vi "沿线段检测边沿点.vi"(6 "开启Overlay":bool, 7 "Edge Options":T4={"Edge Polarity"=0, "Kernel Size"=5, "Width"=11, "Minimum Edge Strength"=10.0, "Interpolation Type"=enum."Bilinear Fixed", "Data Processing Method"=enum."Average"} {"Edge Polarity" items=["All Edges", "Rising Edges", "Falling Edges"]; "Minimum Edge Strength" format="%.2f"; "Width" step=2; "Kernel Size" step=2}, 8 "error in (no error)":errorcluster, 9 "有效":bool, 10 "Caliper Results (Bisect_Slot)":sgl[][](array[numeric]) format="%.2f", 11 "Image":T1) -> (0 "error out":errorcluster, 2 "Edge Information":T3[](array[typedef]) {"Distance (Real-World)" format="%.2f"; "Location (Real-World)"."Y" format="%.2g"; "Location (Real-World)"."X" format="%.2f"; "Noise" format="%.2f"; "Location (Pixel)"."Y" format="%.2g"; "Location (Pixel)"."X" format="%.2f"; "Strength" format="%.2f"; "Distance (Pixel)" format="%.2f"}, 3 "Image Out":T1)   [LabVIEW 2015]
uses:
  <vilib>/vision/Measure.llb/Edge Options.ctl
  <vilib>/vision/Measure.llb/Edge Polarity.ctl
  <vilib>/vision/Measure.llb/Edge New.ctl
  <vilib>/vision/Image Controls.llb/IMAQ Image.ctl
  <vilib>/vision/NI_Vision_Development_Module.lvlib
panel:
  in  "检测线段":T2 {"Start X" scale=0.0..1024.0; "End X" scale=0.0..1024.0}
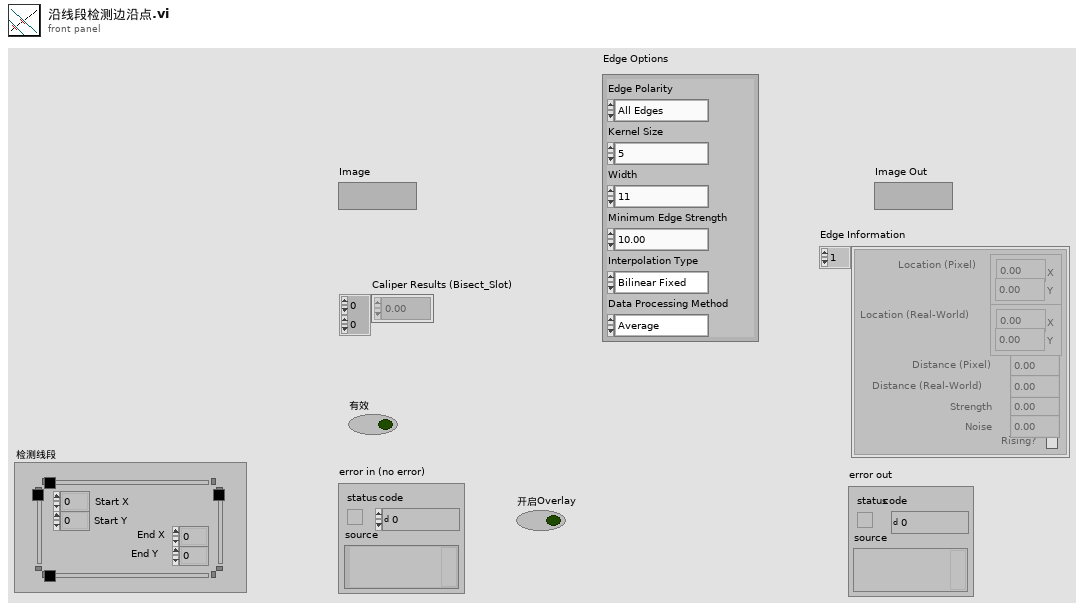
[diagram p1: front panel]
types:
  T1 = typedef "IMAQ Image.ctl" = refnum<image>
  T2 = typedef "IMAQ Line" = cluster{"Start X":i32, "Start Y":i32, "End X":i32, "End Y":i32}
  T3 = typedef "Edge New.ctl" = cluster{"Location (Pixel)":cluster{"X":sgl, "Y":sgl}, "Location (Real-World)":cluster{"X":sgl, "Y":sgl}, "Distance (Pixel)":dbl, "Distance (Real-World)":dbl, "Strength":dbl, "Noise":dbl, "Rising?":bool}
  T4 = typedef "Edge Options.ctl" = cluster{"Edge Polarity":T5, "Kernel Size":u32, "Width":u32, "Minimum Edge Strength":sgl, "Interpolation Type":enum32{"Zero Order", "Bilinear", "Quadratic", "Cubic", "Bilinear Fixed"}, "Data Processing Method":enum32{"Average", "Median"}}
  T5 = typedef "Edge Polarity.ctl" = u32
  T6 = typedef "ROI Descriptor" = cluster{"Global Rectangle":i32[], "Contours":cluster{"ID":enum32{"External", "Internal"}, "Type":u32, "Coordinates":i32[]}[]}
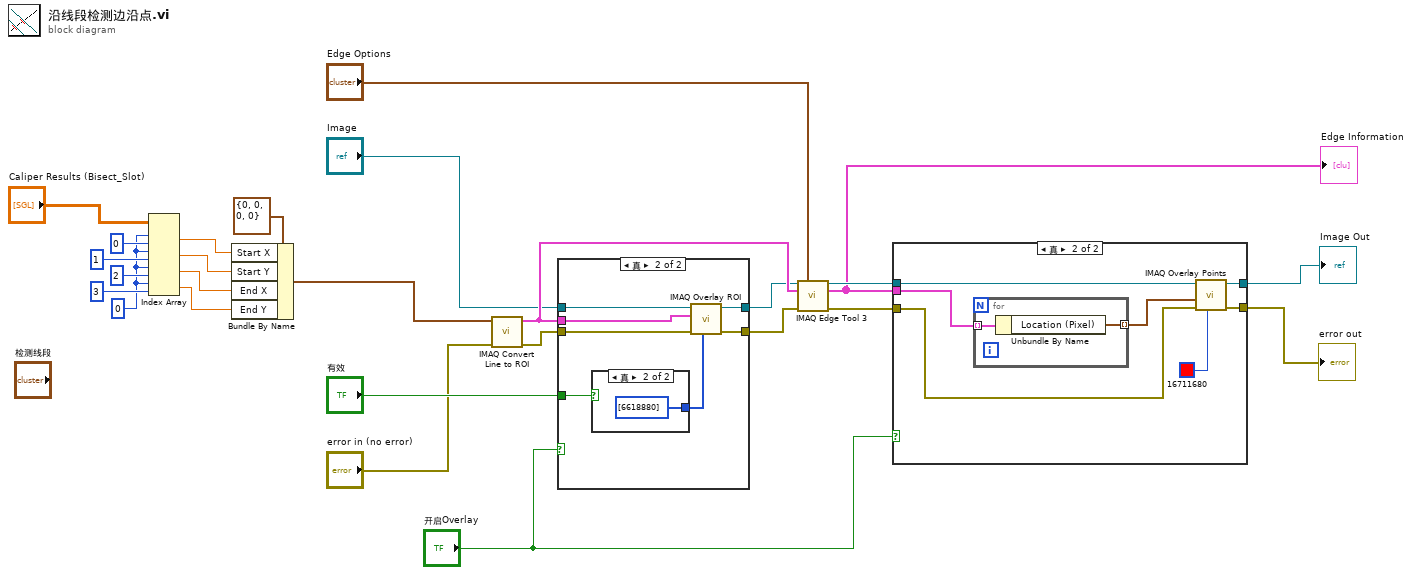
[diagram p0: block diagram]
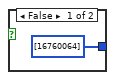
[diagram p4: hidden frame]
diagram:
  w3 = 0 ("索引 (行)")
  n1 = Index Array(array="Caliper Results (Bisect_Slot)", index (row) #1=w3, index (col) #1=0 ("禁用的索引 (列)"), index (row) #2=w3, index (col) #2=1 ("禁用的索引 (列)"), index (row) #3=w3, index (col) #3=2 ("禁用的索引 (列)"), index (row) #4=w3, index (col) #4=3 ("禁用的索引 (列)")) -> (element #1=w8:sgl, element #2=w9:sgl, element #3=w10:sgl, element #4=w11:sgl)
  n2 = Bundle By Name(cluster=T2 {"Start X"=0, "Start Y"=0, "End X"=0, "End Y"=0} ("Line"), "Start X"=w8, "Start Y"=w9, "End X"=w10, "End Y"=w11) -> (w2:T2)
  n3 = call "IMAQ Convert Line to ROI"("error in (no error)"="error in (no error)", "Line"=w2) -> ("error out"=w24:errorcluster, "ROI Descriptor"=w26:T6)  [unwired: 7 in]
  n4 = case shown="真" "开启Overlay" {
    tunnel: w26 -> [_ w34]
    tunnel: [w27 w33] -> w25
    tunnel: w24 -> [w28 w32]
    tunnel: [w28 w31] -> w23
    tunnel: "有效" -> [_ w30]
    tunnel: "Image" -> [w27 w29]
    frame False {
    }
    frame True {
      n5 = case shown="真" w30 {
        tunnel: [u32[] [16760064] ("Colors (Green)") u32[] [6618880] ("Colors (Green)")] -> w35
        frame False {
        }
        frame True {
        }
      }
      n6 = call "IMAQ Overlay ROI"("Colors (Green)"=w35, "error in (no error)"=w32, "ROI Descriptor"=w34, "Image"=w29) -> ("error out"=w31:errorcluster, "Image Out"=w33:T1)  [unwired: 6 in]
    }
  }
  n7 = call "IMAQ Edge Tool 3"("Image"=w25, "Edge Options"="Edge Options", "ROI Descriptor"=w26, "error in (no error)"=w23) -> ("Image (duplicate)"=w21:T1, "Edge Information"=w14:T3[], "error out"=w17:errorcluster)  [unwired: 7 in, 2 out]
  "Edge Information" <- w14
  n8 = case shown="真" "开启Overlay" {
    tunnel: w21 -> [w39 w46]
    tunnel: [w38 w43] -> w18
    tunnel: w17 -> [w38 w42]
    tunnel: [w39 w41] -> w16
    tunnel: w14 -> [_ w40]
    frame False {
    }
    frame True {
      n9 = for {
        tunnel: w40 -> [w48] mode=indexing
        tunnel: [w47] -> w45 mode=indexing
        n10 = Unbundle By Name(w48) -> ("Location (Pixel)"=w47:cluster{"X":sgl, "Y":sgl})
      }
      n11 = call "IMAQ Overlay Points"("Color"=u32 16711680, "error in (no error)"=w42, "Array of Points"=w45, "Image"=w46) -> ("error out"=w43:errorcluster, "Image Out"=w41:T1)  [unwired: 6 in]
    }
  }
  "error out" <- w18
  "Image Out" <- w16
